vi "arthmetic.vi"(2 "Numeric 2":dbl, 3 "operator":string, 4 "Numeric":dbl) -> (1 "String 2":string)   [LabVIEW 2015]
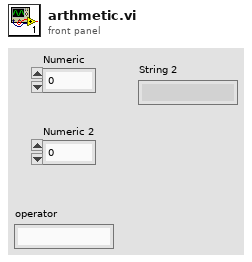
[diagram p1: front panel]
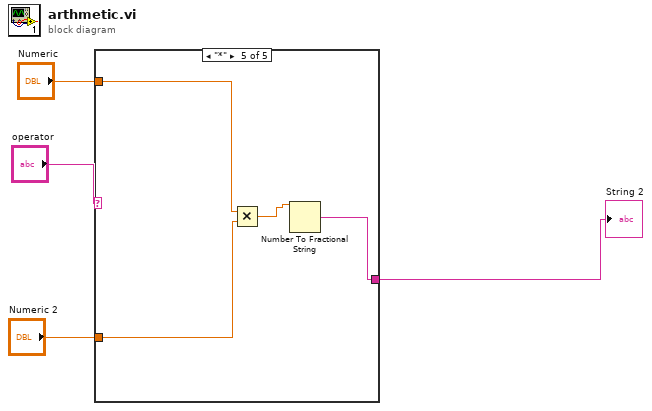
[diagram p0: block diagram]
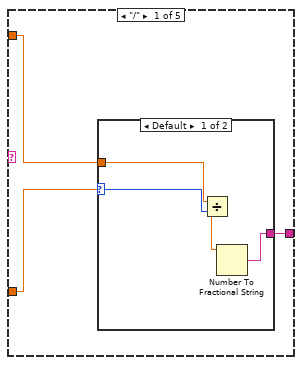
[diagram p2: hidden frame]
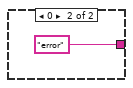
[diagram p3: hidden frame]
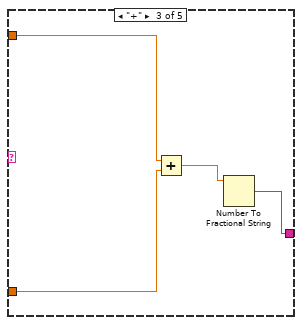
[diagram p5: hidden frame]
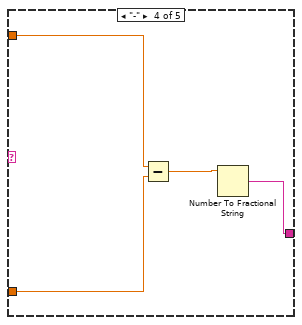
[diagram p6: hidden frame]
diagram:
  n1 = case shown="\"*\"" "operator" {
    selector: "operator" -> [_ w13 _ _ _]
    tunnel: "Numeric" -> [w7 _ w17 w21 w25]
    tunnel: "Numeric 2" -> [w6 _ w16 w20 w24]
    tunnel: [w5 w13 w14 w18 w22] -> w1
    frame "/" {
      n2 = case shown="Default" w6 {
        selector: w6 -> [w10 _]
        tunnel: w7 -> [w11 _]
        tunnel: [w8 "error"] -> w5
        frame Default {
          n3 = Divide(x=w11, y=w10) -> (x/y=w9:dbl)
          n4 = Number To Fractional String(number=w9) -> (F-format string=w8:string)  [unwired: 3 in]
        }
        frame 0 {
        }
      }
    }
    frame Default {
    }
    frame "+" {
      n5 = Add(x=w17, y=w16) -> (x+y=w15:dbl)
      n6 = Number To Fractional String(number=w15) -> (F-format string=w14:string)  [unwired: 3 in]
    }
    frame "-" {
      n7 = Subtract(x=w21, y=w20) -> (x-y=w19:dbl)
      n8 = Number To Fractional String(number=w19) -> (F-format string=w18:string)  [unwired: 3 in]
    }
    frame "*" {
      n9 = Multiply(x=w25, y=w24) -> (x*y=w23:dbl)
      n10 = Number To Fractional String(number=w23) -> (F-format string=w22:string)  [unwired: 3 in]
    }
  }
  "String 2" <- w1
